vi "Blusroutine.vi"() -> ()   [LabVIEW 2021]
uses:
  Global_Variables.vi
panel:
  out "Servo Y angle":dbl
  out "Servo X angle":dbl
  out "Coordinaten":dbl[](array[numeric])
  in  "Gebruik testwaarden":bool
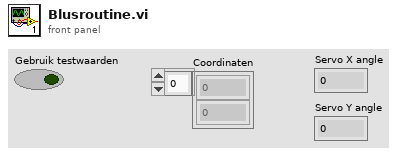
[diagram p1: front panel]
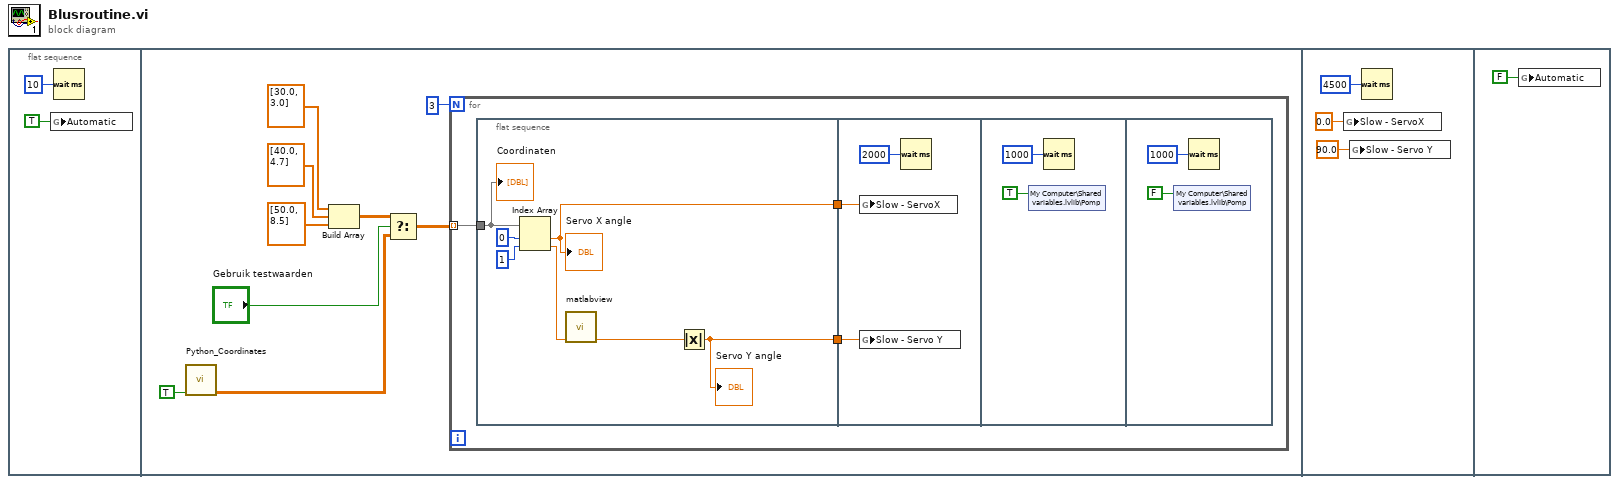
[diagram p0: block diagram]
diagram:
  n1 = flat-sequence {
    frame #0 {
      n2 = global write "Global_Variables.vi" "Automatic"(TRUE) -> ()
      n3 = Wait (ms)(milliseconds to wait=u32 10) -> ()  [unwired: 1 out]
    }
    frame #1 {
      n4 = call "Python_Coordinates.vi"("Angle and distance"=TRUE) -> ("Coordinates"=w4:dbl[][])  [unwired: 10 in]
      n5 = Build Array(dbl[] [30.0, 3.0] ("array"), dbl[] [40.0, 4.7] ("array"), dbl[] [50.0, 8.5] ("array")) -> (w7:dbl[][])
      n6 = Select(t=w7, s="Gebruik testwaarden", f=w4) -> (s? t:f=w6:dbl[][])
      n7 = for {
        N: 3 -> [_]
        tunnel: w6 -> [w12] mode=indexing
        n8 = flat-sequence {
          tunnel: [w16] -> w14
          tunnel: [w19] -> w13
          tunnel: w12 -> [w17]
          tunnel: w14 -> [w22]
          tunnel: w13 -> [w23]
          frame #0 {
            n9 = Index Array(array=w17, index #1=0 ("index"), index #2=1 ("index")) -> (element #1=w16:dbl, element #2=w15:dbl)
            "Servo X angle" <- w16
            n10 = call "matlabview.vi"("Dist"=w15) -> ("Theta_graden"=w20:dbl)  [unwired: 10 in]
            n11 = Absolute Value(x=w20) -> (abs(x)=w19:dbl)
            "Servo Y angle" <- w19
            "Coordinaten" <- w17
          }
          frame #1 {
            n12 = global write "Global_Variables.vi" "Slow - ServoX"(w22) -> ()
            n13 = global write "Global_Variables.vi" "Slow - Servo Y"(w23) -> ()
            n14 = Wait (ms)(milliseconds to wait=u32 2000) -> ()  [unwired: 1 out]
          }
          frame #2 {
            n15 = shared-variable "My Computer\\Shared variables.lvlib\\Pomp"(TRUE ("Pomp")) -> ()  [unwired: 1 in, 1 out]
            n16 = Wait (ms)(milliseconds to wait=u32 1000) -> ()  [unwired: 1 out]
          }
          frame #3 {
            n17 = shared-variable "My Computer\\Shared variables.lvlib\\Pomp"(FALSE ("Pomp")) -> ()  [unwired: 1 in, 1 out]
            n18 = Wait (ms)(milliseconds to wait=u32 1000) -> ()  [unwired: 1 out]
          }
        }
      }
    }
    frame #2 {
      n19 = global write "Global_Variables.vi" "Slow - ServoX"(0.0 ("Servo Y")) -> ()
      n20 = global write "Global_Variables.vi" "Slow - Servo Y"(90.0 ("Servo X")) -> ()
      n21 = Wait (ms)(milliseconds to wait=u32 4500) -> ()  [unwired: 1 out]
    }
    frame #3 {
      n22 = global write "Global_Variables.vi" "Automatic"(FALSE) -> ()
    }
  }
